vi "TCP Read Data.vi"(4 "error in (no error)":errorcluster, 5 "Timeout (25000 ms)":i32=25000, 7 "connection ID":refnum<k5>) -> (0 "error out":errorcluster, 1 "Timeout?":bool, 2 "Flat Data":string, 3 "dup connection ID":refnum<k5>)   [LabVIEW 2011]
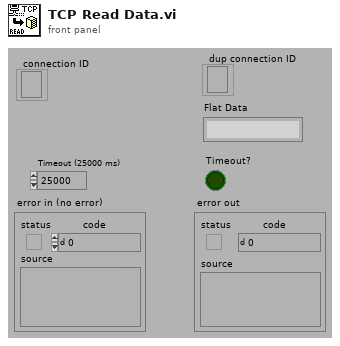
[diagram p1: front panel]
types:
  T1 = enum16{"Standard", "Buffered", "CRLF", "Immediate"}
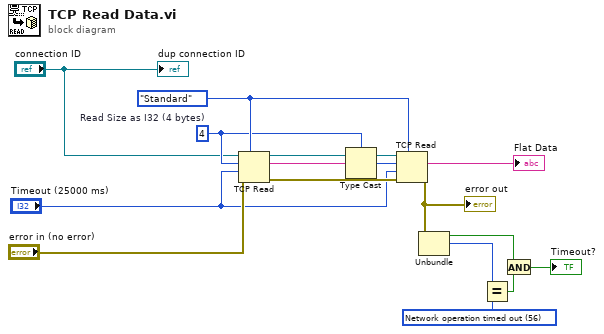
[diagram p0: block diagram]
diagram:
  w8 = 56 items=["No error", "Argument error", "Memory is full", "Out of zone", "End of file", "File already open", "Generic file I/O error", "File not found", "File permission error", "Disk is full", "Duplicate path", "Too many files open", "System feature not enabled", "Resource file not found", "Cannot add resource", "Resource not found", "Image not found", "Image memory error", "Pen does not exist", "Config type invalid", "Config token not found", "Config parse error", "Config memory error", "Bad external code format", "Bad external code offset", "External code not present", "Null window", "Destroy window error", "Null menu", "Print aborted", "Bad print record", "Print driver error", "Windows error during printing", "Memory error during printing", "Print dialog error", "Generic print error", "Invalid device refnum", "Device not found", "Device parameter error", "Device unit error", "Cannot open device", "Device call aborted", "Generic error", "Cancelled by user", "Object ID too low", "Object ID too high", "Object not in heap", "Unknown heap", "Unknown object (invalid DefProc)", "Unknown object (DefProc not in table)", "Message out of range", "Invalid (null) method", "Unknown message", "Manager call not supported", "Bad address", "Network operation in progress", "Network operation timed out", "Connection is busy", "Network attribute not supported", "Network error", "Address in use", "System out of memory", "Connection aborted", "Connection refused", "Not connected", "Already connected", "Connection closed", "Initialization error (interapplication manager)", "Bad occurrence", "Wait on unbound occurrence handler", "Occurrence queue overflow", "Datalog type conflict", "Unused", "Unrecognized type (interapplication manager)", "Memory corrupt", "Failed to make temporary DLL", "Old CIN version", "Drag socket not found", "Failed to load drop-object", "Failed to register OLE object", "Failed to release OLE object", "Format specifier type mismatch", "Unknown format specifier", "Too few format specifiers", "Too many format specifiers", "Scan failed", "Newer CIN version", "Error converting to variant", "Runtime menu error", "Password tampered", "Variant attribute not found", "Incompatible variant data type", "Event data is not available", "Event Store is not present", "Occurrence is not found", "Event Queue is not created", "Event info is not available", "Refnum passed is NULL", "Error retrieving Class GUID", "Error retrieving CoClass GUID", "Error retrieving TypeLib GUID.", "Bad built application magic bytes.", "Specific driver is different from the specific driver associated with the Logical Name.", "There is no session opened to the class driver.", "Max Error", "MAX - Error with config objects", "MAX - Error loading configuration", "MAX - Group not supported"]
  w14 = 4  # Read Size as I32 (4 bytes)
  w16 = T1."Standard" ("mode (standard)")
  n1 = TCP Read(connection ID="connection ID", bytes to read=w14, error in (no error)="error in (no error)", 7:w16, 9:"Timeout (25000 ms)") -> (connection ID out=w12:refnum<k5>, data out=w2:string, error out=w13:errorcluster)
  n2 = Type Cast(type=w14, x=w2) -> (*(type *) &x=w15:i32)
  n3 = TCP Read(connection ID=w12, bytes to read=w15, error in (no error)=w13, 7:w16, 9:"Timeout (25000 ms)") -> (data out=→"Flat Data":string, error out=w6:errorcluster)  [unwired: 1 out]
  "error out" <- w6
  n4 = Unbundle(w6) -> ("status"=w5:bool, "code"=w4:i32)  [unwired: 1 out]
  n5 = Equal?(x=w4, y=w8) -> (x = y?=w7:bool)
  n6 = And(x=w5, y=w7) -> (x .and. y?=→"Timeout?":bool)
  "dup connection ID" <- "connection ID"
